vi "App - analyze RUS V6.vi"() -> ()   [LabVIEW 2018] (continued)
"temperature str"="184.42600", "file path"=path "D:/Data/Ultrasound/LSCO/LSCO22__130814c/5_Cooling_2nd_try/September_2014/091614/184.42600K_500_2500_2.10000V_0.00000T_Sep16-2014__15-25-55_001_091614.bin", "last mod"=timestamp(3493740355 s since 1904-01-01), "file name str"="D:\\Data\\Ultrasound\\LSCO\\LSCO22__130814c\\5_Cooling_2nd_try\\September_2014\\091614\\184.42600K_500_2500_2.10000V_0.00000T_Sep16-2014__15-25-55_001_091614.bin", "mod time(min)"=58229005.916666664, "file format"=enum."binary", "power(V)"=2.1, "Magn Field(T) "=0.0}, {"temperature"=184.132, "temperature str"="184.13200", "file path"=path "D:/Data/Ultrasound/LSCO/LSCO22__130814c/5_Cooling_2nd_try/September_2014/091614/184.13200K_500_2500_2.10000V_0.00000T_Sep16-2014__15-27-14_001_091614.bin", "last mod"=timestamp(3493740434 s since 1904-01-01), "file name str"="D:\\Data\\Ultrasound\\LSCO\\LSCO22__130814c\\5_Cooling_2nd_try\\September_2014\\091614\\184.13200K_500_2500_2.10000V_0.00000T_Sep16-2014__15-27-14_001_091614.bin", "mod time(min)"=58229007.233333334, "file format"=enum."binary", "power(V)"=2.1, "Magn Field(T) "=0.0}, {"temperature"=183.85, "temperature str"="183.85000", "file path"=path "D:/Data/Ultrasound/LSCO/LSCO22__130814c/5_Cooling_2nd_try/September_2014/091614/183.85000K_500_2500_2.10000V_0.00000T_Sep16-2014__15-28-33_001_091614.bin", "last mod"=timestamp(3493740513 s since 1904-01-01), "file name str"="D:\\Data\\Ultrasound\\LSCO\\LSCO22__130814c\\5_Cooling_2nd_try\\September_2014\\091614\\183.85000K_500_2500_2.10000V_0.00000T_Sep16-2014__15-28-33_001_091614.bin", "mod time(min)"=58229008.55, "file format"=enum."binary", "power(V)"=2.1, "Magn Field(T) "=0.0}, {"temperature"=183.537, "temperature str"="183.53700", "file path"=path "D:/Data/Ultrasound/LSCO/LSCO22__130814c/5_Cooling_2nd_try/September_2014/091614/183.53700K_500_2500_2.10000V_0.00000T_Sep16-2014__15-29-53_001_091614.bin", "last mod"=timestamp(3493740593 s since 1904-01-01), "file name str"="D:\\Data\\Ultrasound\\LSCO\\LSCO22__130814c\\5_Cooling_2nd_try\\September_2014\\091614\\183.53700K_500_2500_2.10000V_0.00000T_Sep16-2014__15-29-53_001_091614.bin", "mod time(min)"=58229009.88333333, "file format"=enum."binary", "power(V)"=2.1, "Magn Field(T) "=0.0}, {"temperature"=183.227, "temperature str"="183.22700", "file path"=path "D:/Data/Ultrasound/LSCO/LSCO22__130814c/5_Cooling_2nd_try/September_2014/091614/183.22700K_500_2500_2.10000V_0.00000T_Sep16-2014__15-31-12_001_091614.bin", "last mod"=timestamp(3493740672 s since 1904-01-01), "file name str"="D:\\Data\\Ultrasound\\LSCO\\LSCO22__130814c\\5_Cooling_2nd_try\\September_2014\\091614\\183.22700K_500_2500_2.10000V_0.00000T_Sep16-2014__15-31-12_001_091614.bin", "mod time(min)"=58229011.2, "file format"=enum."binary", "power(V)"=2.1, "Magn Field(T) "=0.0}, {"temperature"=182.898, "temperature str"="182.89800", "file path"=path "D:/Data/Ultrasound/LSCO/LSCO22__130814c/5_Cooling_2nd_try/September_2014/091614/182.89800K_500_2500_2.10000V_0.00000T_Sep16-2014__15-32-31_001_091614.bin", "last mod"=timestamp(3493740751 s since 1904-01-01), "file name str"="D:\\Data\\Ultrasound\\LSCO\\LSCO22__130814c\\5_Cooling_2nd_try\\September_2014\\091614\\182.89800K_500_2500_2.10000V_0.00000T_Sep16-2014__15-32-31_001_091614.bin", "mod time(min)"=58229012.516666666, "file format"=enum."binary", "power(V)"=2.1, "Magn Field(T) "=0.0}, {"temperature"=182.567, "temperature str"="182.56700", "file path"=path "D:/Data/Ultrasound/LSCO/LSCO22__130814c/5_Cooling_2nd_try/September_2014/091614/182.56700K_500_2500_2.10000V_0.00000T_Sep16-2014__15-33-51_001_091614.bin", "last mod"=timestamp(3493740831 s since 1904-01-01), "file name str"="D:\\Data\\Ultrasound\\LSCO\\LSCO22__130814c\\5_Cooling_2nd_try\\September_2014\\091614\\182.56700K_500_2500_2.10000V_0.00000T_Sep16-2014__15-33-51_001_091614.bin", "mod time(min)"=58229013.85, "file format"=enum."binary", "power(V)"=2.1, "Magn Field(T) "=0.0}, {"temperature"=182.25, "temperature str"="182.25000", "file path"=path "D:/Data/Ultrasound/LSCO/LSCO22__130814c/5_Cooling_2nd_try/September_2014/091614/182.25000K_500_2500_2.10000V_0.00000T_Sep16-2014__15-35-10_001_091614.bin", "last mod"=timestamp(3493740910 s since 1904-01-01), "file name str"="D:\\Data\\Ultrasound\\LSCO\\LSCO22__130814c\\5_Cooling_2nd_try\\September_2014\\091614\\182.25000K_500_2500_2.10000V_0.00000T_Sep16-2014__15-35-10_001_091614.bin", "mod time(min)"=58229015.166666664, "file format"=enum."binary", "power(V)"=2.1, "Magn Field(T) "=0.0}, {"temperature"=181.923, "temperature str"="181.92300", "file path"=path "D:/Data/Ultrasound/LSCO/LSCO22__130814c/5_Cooling_2nd_try/September_2014/091614/181.92300K_500_2500_2.10000V_0.00000T_Sep16-2014__15-36-30_001_091614.bin", "last mod"=timestamp(3493740990 s since 1904-01-01), "file name str"="D:\\Data\\Ultrasound\\LSCO\\LSCO22__130814c\\5_Cooling_2nd_try\\September_2014\\091614\\181.92300K_500_2500_2.10000V_0.00000T_Sep16-2014__15-36-30_001_091614.bin", "mod time(min)"=58229016.5, "file format"=enum."binary", "power(V)"=2.1, "Magn Field(T) "=0.0}, {"temperature"=181.605, "temperature str"="181.60500", "file path"=path "D:/Data/Ultrasound/LSCO/LSCO22__130814c/5_Cooling_2nd_try/September_2014/091614/181.60500K_500_2500_2.10000V_0.00000T_Sep16-2014__15-37-49_001_091614.bin", "last mod"=timestamp(3493741069 s since 1904-01-01), "file name str"="D:\\Data\\Ultrasound\\LSCO\\LSCO22__130814c\\5_Cooling_2nd_try\\September_2014\\091614\\181.60500K_500_2500_2.10000V_0.00000T_Sep16-2014__15-37-49_001_091614.bin", "mod time(min)"=58229017.81666667, "file format"=enum."binary", "power(V)"=2.1, "Magn Field(T) "=0.0}, {"temperature"=181.283, "temperature str"="181.28300", "file path"=path "D:/Data/Ultrasound/LSCO/LSCO22__130814c/5_Cooling_2nd_try/September_2014/091614/181.28300K_500_2500_2.10000V_0.00000T_Sep16-2014__15-39-08_001_091614.bin", "last mod"=timestamp(3493741148 s since 1904-01-01), "file name str"="D:\\Data\\Ultrasound\\LSCO\\LSCO22__130814c\\5_Cooling_2nd_try\\September_2014\\091614\\181.28300K_500_2500_2.10000V_0.00000T_Sep16-2014__15-39-08_001_091614.bin", "mod time(min)"=58229019.13333333, "file format"=enum."binary", "power(V)"=2.1, "Magn Field(T) "=0.0}, {"temperature"=180.967, "temperature str"="180.96700", "file path"=path "D:/Data/Ultrasound/LSCO/LSCO22__130814c/5_Cooling_2nd_try/September_2014/091614/180.96700K_500_2500_2.10000V_0.00000T_Sep16-2014__15-40-28_001_091614.bin", "last mod"=timestamp(3493741228 s since 1904-01-01), "file name str"="D:\\Data\\Ultrasound\\LSCO\\LSCO22__130814c\\5_Cooling_2nd_try\\September_2014\\091614\\180.96700K_500_2500_2.10000V_0.00000T_Sep16-2014__15-40-28_001_091614.bin", "mod time(min)"=58229020.46666667, "file format"=enum."binary", "power(V)"=2.1, "Magn Field(T) "=0.0}, {"temperature"=180.662, "temperature str"="180.66200", "file path"=path "D:/Data/Ultrasound/LSCO/LSCO22__130814c/5_Cooling_2nd_try/September_2014/091614/180.66200K_500_2500_2.10000V_0.00000T_Sep16-2014__15-41-47_001_091614.bin", "last mod"=timestamp(3493741307 s since 1904-01-01), "file name str"="D:\\Data\\Ultrasound\\LSCO\\LSCO22__130814c\\5_Cooling_2nd_try\\September_2014\\091614\\180.66200K_500_2500_2.10000V_0.00000T_Sep16-2014__15-41-47_001_091614.bin", "mod time(min)"=58229021.78333333, "file format"=enum."binary", "power(V)"=2.1, "Magn Field(T) "=0.0}, {"temperature"=180.335, "temperature str"="180.33500", "file path"=path "D:/Data/Ultrasound/LSCO/LSCO22__130814c/5_Cooling_2nd_try/September_2014/091614/180.33500K_500_2500_2.10000V_0.00000T_Sep16-2014__15-43-06_001_091614.bin", "last mod"=timestamp(3493741386 s since 1904-01-01), "file name str"="D:\\Data\\Ultrasound\\LSCO\\LSCO22__130814c\\5_Cooling_2nd_try\\September_2014\\091614\\180.33500K_500_2500_2.10000V_0.00000T_Sep16-2014__15-43-06_001_091614.bin", "mod time(min)"=58229023.1, "file format"=enum."binary", "power(V)"=2.1, "Magn Field(T) "=0.0}, {"temperature"=180.012, "temperature str"="180.01200", "file path"=path "D:/Data/Ultrasound/LSCO/LSCO22__130814c/5_Cooling_2nd_try/September_2014/091614/180.01200K_500_2500_2.10000V_0.00000T_Sep16-2014__15-44-26_001_091614.bin", "last mod"=timestamp(3493741466 s since 1904-01-01), "file name str"="D:\\Data\\Ultrasound\\LSCO\\LSCO22__130814c\\5_Cooling_2nd_try\\September_2014\\091614\\180.01200K_500_2500_2.10000V_0.00000T_Sep16-2014__15-44-26_001_091614.bin", "mod time(min)"=58229024.43333333, "file format"=enum."binary", "power(V)"=2.1, "Magn Field(T) "=0.0}, {"temperature"=179.664, "temperature str"="179.66400", "file path"=path "D:/Data/Ultrasound/LSCO/LSCO22__130814c/5_Cooling_2nd_try/September_2014/091614/179.66400K_500_2500_2.10000V_0.00000T_Sep16-2014__15-45-45_001_091614.bin", "last mod"=timestamp(3493741545 s since 1904-01-01), "file name str"="D:\\Data\\Ultrasound\\LSCO\\LSCO22__130814c\\5_Cooling_2nd_try\\September_2014\\091614\\179.66400K_500_2500_2.10000V_0.00000T_Sep16-2014__15-45-45_001_091614.bin", "mod time(min)"=58229025.75, "file format"=enum."binary", "power(V)"=2.1, "Magn Field(T) "=0.0}, {"temperature"=179.311, "temperature str"="179.31100", "file path"=path "D:/Data/Ultrasound/LSCO/LSCO22__130814c/5_Cooling_2nd_try/September_2014/091614/179.31100K_500_2500_2.10000V_0.00000T_Sep16-2014__15-47-05_001_091614.bin", "last mod"=timestamp(3493741625 s since 1904-01-01), "file name str"="D:\\Data\\Ultrasound\\LSCO\\LSCO22__130814c\\5_Cooling_2nd_try\\September_2014\\091614\\179.31100K_500_2500_2.10000V_0.00000T_Sep16-2014__15-47-05_001_091614.bin", "mod time(min)"=58229027.083333336, "file format"=enum."binary", "power(V)"=2.1, "Magn Field(T) "=0.0}, {"temperature"=178.96, "temperature str"="178.96000", "file path"=path "D:/Data/Ultrasound/LSCO/LSCO22__130814c/5_Cooling_2nd_try/September_2014/091614/178.96000K_500_2500_2.10000V_0.00000T_Sep16-2014__15-48-24_001_091614.bin", "last mod"=timestamp(3493741704 s since 1904-01-01), "file name str"="D:\\Data\\Ultrasound\\LSCO\\LSCO22__130814c\\5_Cooling_2nd_try\\September_2014\\091614\\178.96000K_500_2500_2.10000V_0.00000T_Sep16-2014__15-48-24_001_091614.bin", "mod time(min)"=58229028.4, "file format"=enum."binary", "power(V)"=2.1, "Magn Field(T) "=0.0}, {"temperature"=178.579, "temperature str"="178.57900", "file path"=path "D:/Data/Ultrasound/LSCO/LSCO22__130814c/5_Cooling_2nd_try/September_2014/091614/178.57900K_500_2500_2.10000V_0.00000T_Sep16-2014__15-49-43_001_091614.bin", "last mod"=timestamp(3493741783 s since 1904-01-01), "file name str"="D:\\Data\\Ultrasound\\LSCO\\LSCO22__130814c\\5_Cooling_2nd_try\\September_2014\\091614\\178.57900K_500_2500_2.10000V_0.00000T_Sep16-2014__15-49-43_001_091614.bin", "mod time(min)"=58229029.71666667, "file format"=enum."binary", "power(V)"=2.1, "Magn Field(T) "=0.0}, {"temperature"=178.21, "temperature str"="178.21000", "file path"=path "D:/Data/Ultrasound/LSCO/LSCO22__130814c/5_Cooling_2nd_try/September_2014/091614/178.21000K_500_2500_2.10000V_0.00000T_Sep16-2014__15-51-03_001_091614.bin", "last mod"=timestamp(3493741863 s since 1904-01-01), "file name str"="D:\\Data\\Ultrasound\\LSCO\\LSCO22__130814c\\5_Cooling_2nd_try\\September_2014\\091614\\178.21000K_500_2500_2.10000V_0.00000T_Sep16-2014__15-51-03_001_091614.bin", "mod time(min)"=58229031.05, "file format"=enum."binary", "power(V)"=2.1, "Magn Field(T) "=0.0}, {"temperature"=177.848, "temperature str"="177.84800", "file path"=path "D:/Data/Ultrasound/LSCO/LSCO22__130814c/5_Cooling_2nd_try/September_2014/091614/177.84800K_500_2500_2.10000V_0.00000T_Sep16-2014__15-52-22_001_091614.bin", "last mod"=timestamp(3493741942 s since 1904-01-01), "file name str"="D:\\Data\\Ultrasound\\LSCO\\LSCO22__130814c\\5_Cooling_2nd_try\\September_2014\\091614\\177.84800K_500_2500_2.10000V_0.00000T_Sep16-2014__15-52-22_001_091614.bin", "mod time(min)"=58229032.36666667, "file format"=enum."binary", "power(V)"=2.1, "Magn Field(T) "=0.0}, {"temperature"=177.556, "temperature str"="177.55600", "file path"=path "D:/Data/Ultrasound/LSCO/LSCO22__130814c/5_Cooling_2nd_try/September_2014/091614/177.55600K_500_2500_2.10000V_0.00000T_Sep16-2014__15-53-41_001_091614.bin", "last mod"=timestamp(3493742021 s since 1904-01-01), "file name str"="D:\\Data\\Ultrasound\\LSCO\\LSCO22__130814c\\5_Cooling_2nd_try\\September_2014\\091614\\177.55600K_500_2500_2.10000V_0.00000T_Sep16-2014__15-53-41_001_091614.bin", "mod time(min)"=58229033.68333333, "file format"=enum."binary", "power(V)"=2.1, "Magn Field(T) "=0.0}, {"temperature"=177.306, "temperature str"="177.30600", "file path"=path "D:/Data/Ultrasound/LSCO/LSCO22__130814c/5_Cooling_2nd_try/September_2014/091614/177.30600K_500_2500_2.10000V_0.00000T_Sep16-2014__15-55-01_001_091614.bin", "last mod"=timestamp(3493742101 s since 1904-01-01), "file name str"="D:\\Data\\Ultrasound\\LSCO\\LSCO22__130814c\\5_Cooling_2nd_try\\September_2014\\091614\\177.30600K_500_2500_2.10000V_0.00000T_Sep16-2014__15-55-01_001_091614.bin", "mod time(min)"=58229035.016666666, "file format"=enum."binary", "power(V)"=2.1, "Magn Field(T) "=0.0}, {"temperature"=177.009, "temperature str"="177.00900", "file path"=path "D:/Data/Ultrasound/LSCO/LSCO22__130814c/5_Cooling_2nd_try/September_2014/091614/177.00900K_500_2500_2.10000V_0.00000T_Sep16-2014__15-56-20_001_091614.bin", "last mod"=timestamp(3493742180 s since 1904-01-01), "file name str"="D:\\Data\\Ultrasound\\LSCO\\LSCO22__130814c\\5_Cooling_2nd_try\\September_2014\\091614\\177.00900K_500_2500_2.10000V_0.00000T_Sep16-2014__15-56-20_001_091614.bin", "mod time(min)"=58229036.333333336, "file format"=enum."binary", "power(V)"=2.1, "Magn Field(T) "=0.0}, {"temperature"=176.677, "temperature str"="176.67700", "file path"=path "D:/Data/Ultrasound/LSCO/LSCO22__130814c/5_Cooling_2nd_try/September_2014/091614/176.67700K_500_2500_2.10000V_0.00000T_Sep16-2014__15-57-39_001_091614.bin", "last mod"=timestamp(3493742259 s since 1904-01-01), "file name str"="D:\\Data\\Ultrasound\\LSCO\\LSCO22__130814c\\5_Cooling_2nd_try\\September_2014\\091614\\176.67700K_500_2500_2.10000V_0.00000T_Sep16-2014__15-57-39_001_091614.bin", "mod time(min)"=58229037.65, "file format"=enum."binary", "power(V)"=2.1, "Magn Field(T) "=0.0}, {"temperature"=176.315, "temperature str"="176.31500", "file path"=path "D:/Data/Ultrasound/LSCO/LSCO22__130814c/5_Cooling_2nd_try/September_2014/091614/176.31500K_500_2500_2.10000V_0.00000T_Sep16-2014__15-58-59_001_091614.bin", "last mod"=timestamp(3493742339 s since 1904-01-01), "file name str"="D:\\Data\\Ultrasound\\LSCO\\LSCO22__130814c\\5_Cooling_2nd_try\\September_2014\\091614\\176.31500K_500_2500_2.10000V_0.00000T_Sep16-2014__15-58-59_001_091614.bin", "mod time(min)"=58229038.983333334, "file format"=enum."binary", "power(V)"=2.1, "Magn Field(T) "=0.0}, {"temperature"=175.963, "temperature str"="175.96300", "file path"=path "D:/Data/Ultrasound/LSCO/LSCO22__130814c/5_Cooling_2nd_try/September_2014/091614/175.96300K_500_2500_2.10000V_0.00000T_Sep16-2014__16-00-18_001_091614.bin", "last mod"=timestamp(3493742418 s since 1904-01-01), "file name str"="D:\\Data\\Ultrasound\\LSCO\\LSCO22__130814c\\5_Cooling_2nd_try\\September_2014\\091614\\175.96300K_500_2500_2.10000V_0.00000T_Sep16-2014__16-00-18_001_091614.bin", "mod time(min)"=58229040.3, "file format"=enum."binary", "power(V)"=2.1, "Magn Field(T) "=0.0}, {"temperature"=175.634, "temperature str"="175.63400", "file path"=path "D:/Data/Ultrasound/LSCO/LSCO22__130814c/5_Cooling_2nd_try/September_2014/091614/175.63400K_500_2500_2.10000V_0.00000T_Sep16-2014__16-01-37_001_091614.bin", "last mod"=timestamp(3493742497 s since 1904-01-01), "file name str"="D:\\Data\\Ultrasound\\LSCO\\LSCO22__130814c\\5_Cooling_2nd_try\\September_2014\\091614\\175.63400K_500_2500_2.10000V_0.00000T_Sep16-2014__16-01-37_001_091614.bin", "mod time(min)"=58229041.61666667, "file format"=enum."binary", "power(V)"=2.1, "Magn Field(T) "=0.0}, {"temperature"=175.302, "temperature str"="175.30200", "file path"=path "D:/Data/Ultrasound/LSCO/LSCO22__130814c/5_Cooling_2nd_try/September_2014/091614/175.30200K_500_2500_2.10000V_0.00000T_Sep16-2014__16-02-57_001_091614.bin", "last mod"=timestamp(3493742577 s since 1904-01-01), "file name str"="D:\\Data\\Ultrasound\\LSCO\\LSCO22__130814c\\5_Cooling_2nd_try\\September_2014\\091614\\175.30200K_500_2500_2.10000V_0.00000T_Sep16-2014__16-02-57_001_091614.bin", "mod time(min)"=58229042.95, "file format"=enum."binary", "power(V)"=2.1, "Magn Field(T) "=0.0}, {"temperature"=174.985, "temperature str"="174.98500", "file path"=path "D:/Data/Ultrasound/LSCO/LSCO22__130814c/5_Cooling_2nd_try/September_2014/091614/174.98500K_500_2500_2.10000V_0.00000T_Sep16-2014__16-04-16_001_091614.bin", "last mod"=timestamp(3493742656 s since 1904-01-01), "file name str"="D:\\Data\\Ultrasound\\LSCO\\LSCO22__130814c\\5_Cooling_2nd_try\\September_2014\\091614\\174.98500K_500_2500_2.10000V_0.00000T_Sep16-2014__16-04-16_001_091614.bin", "mod time(min)"=58229044.266666666, "file format"=enum."binary", "power(V)"=2.1, "Magn Field(T) "=0.0}, {"temperature"=174.654, "temperature str"="174.65400", "file path"=path "D:/Data/Ultrasound/LSCO/LSCO22__130814c/5_Cooling_2nd_try/September_2014/091614/174.65400K_500_2500_2.10000V_0.00000T_Sep16-2014__16-05-35_001_091614.bin", "last mod"=timestamp(3493742735 s since 1904-01-01), "file name str"="D:\\Data\\Ultrasound\\LSCO\\LSCO22__130814c\\5_Cooling_2nd_try\\September_2014\\091614\\174.65400K_500_2500_2.10000V_0.00000T_Sep16-2014__16-05-35_001_091614.bin", "mod time(min)"=58229045.583333336, "file format"=enum."binary", "power(V)"=2.1, "Magn Field(T) "=0.0}, {"temperature"=174.316, "temperature str"="174.31600", "file path"=path "D:/Data/Ultrasound/LSCO/LSCO22__130814c/5_Cooling_2nd_try/September_2014/091614/174.31600K_500_2500_2.10000V_0.00000T_Sep16-2014__16-06-55_001_091614.bin", "last mod"=timestamp(3493742815 s since 1904-01-01), "file name str"="D:\\Data\\Ultrasound\\LSCO\\LSCO22__130814c\\5_Cooling_2nd_try\\September_2014\\091614\\174.31600K_500_2500_2.10000V_0.00000T_Sep16-2014__16-06-55_001_091614.bin", "mod time(min)"=58229046.916666664, "file format"=enum."binary", "power(V)"=2.1, "Magn Field(T) "=0.0}, {"temperature"=173.984, "temperature str"="173.98400", "file path"=path "D:/Data/Ultrasound/LSCO/LSCO22__130814c/5_Cooling_2nd_try/September_2014/091614/173.98400K_500_2500_2.10000V_0.00000T_Sep16-2014__16-08-14_001_091614.bin", "last mod"=timestamp(3493742894 s since 1904-01-01), "file name str"="D:\\Data\\Ultrasound\\LSCO\\LSCO22__130814c\\5_Cooling_2nd_try\\September_2014\\091614\\173.98400K_500_2500_2.10000V_0.00000T_Sep16-2014__16-08-14_001_091614.bin", "mod time(min)"=58229048.233333334, "file format"=enum."binary", "power(V)"=2.1, "Magn Field(T) "=0.0}, {"temperature"=173.642, "temperature str"="173.64200", "file path"=path "D:/Data/Ultrasound/LSCO/LSCO22__130814c/5_Cooling_2nd_try/September_2014/091614/173.64200K_500_2500_2.10000V_0.00000T_Sep16-2014__16-09-33_001_091614.bin", "last mod"=timestamp(3493742973 s since 1904-01-01), "file name str"="D:\\Data\\Ultrasound\\LSCO\\LSCO22__130814c\\5_Cooling_2nd_try\\September_2014\\091614\\173.64200K_500_2500_2.10000V_0.00000T_Sep16-2014__16-09-33_001_091614.bin", "mod time(min)"=58229049.55, "file format"=enum."binary", "power(V)"=2.1, "Magn Field(T) "=0.0}, {"temperature"=173.314, "temperature str"="173.31400", "file path"=path "D:/Data/Ultrasound/LSCO/LSCO22__130814c/5_Cooling_2nd_try/September_2014/091614/173.31400K_500_2500_2.10000V_0.00000T_Sep16-2014__16-10-53_001_091614.bin", "last mod"=timestamp(3493743053 s since 1904-01-01), "file name str"="D:\\Data\\Ultrasound\\LSCO\\LSCO22__130814c\\5_Cooling_2nd_try\\September_2014\\091614\\173.31400K_500_2500_2.10000V_0.00000T_Sep16-2014__16-10-53_001_091614.bin", "mod time(min)"=58229050.88333333, "file format"=enum."binary", "power(V)"=2.1, "Magn Field(T) "=0.0}, {"temperature"=172.974, "temperature str"="172.97400", "file path"=path "D:/Data/Ultrasound/LSCO/LSCO22__130814c/5_Cooling_2nd_try/September_2014/091614/172.97400K_500_2500_2.10000V_0.00000T_Sep16-2014__16-12-12_001_091614.bin", "last mod"=timestamp(3493743132 s since 1904-01-01), "file name str"="D:\\Data\\Ultrasound\\LSCO\\LSCO22__130814c\\5_Cooling_2nd_try\\September_2014\\091614\\172.97400K_500_2500_2.10000V_0.00000T_Sep16-2014__16-12-12_001_091614.bin", "mod time(min)"=58229052.2, "file format"=enum."binary", "power(V)"=2.1, "Magn Field(T) "=0.0}, {"temperature"=172.632, "temperature str"="172.63200", "file path"=path "D:/Data/Ultrasound/LSCO/LSCO22__130814c/5_Cooling_2nd_try/September_2014/091614/172.63200K_500_2500_2.10000V_0.00000T_Sep16-2014__16-13-31_001_091614.bin", "last mod"=timestamp(3493743211 s since 1904-01-01), "file name str"="D:\\Data\\Ultrasound\\LSCO\\LSCO22__130814c\\5_Cooling_2nd_try\\September_2014\\091614\\172.63200K_500_2500_2.10000V_0.00000T_Sep16-2014__16-13-31_001_091614.bin", "mod time(min)"=58229053.516666666, "file format"=enum."binary", "power(V)"=2.1, "Magn Field(T) "=0.0}, {"temperature"=172.303, "temperature str"="172.30300", "file path"=path "D:/Data/Ultrasound/LSCO/LSCO22__130814c/5_Cooling_2nd_try/September_2014/091614/172.30300K_500_2500_2.10000V_0.00000T_Sep16-2014__16-14-51_001_091614.bin", "last mod"=timestamp(3493743291 s since 1904-01-01), "file name str"="D:\\Data\\Ultrasound\\LSCO\\LSCO22__130814c\\5_Cooling_2nd_try\\September_2014\\091614\\172.30300K_500_2500_2.10000V_0.00000T_Sep16-2014__16-14-51_001_091614.bin", "mod time(min)"=58229054.85, "file format"=enum."binary", "power(V)"=2.1, "Magn Field(T) "=0.0}, {"temperature"=171.947, "temperature str"="171.94700", "file path"=path "D:/Data/Ultrasound/LSCO/LSCO22__130814c/5_Cooling_2nd_try/September_2014/091614/171.94700K_500_2500_2.10000V_0.00000T_Sep16-2014__16-16-10_001_091614.bin", "last mod"=timestamp(3493743370 s since 1904-01-01), "file name str"="D:\\Data\\Ultrasound\\LSCO\\LSCO22__130814c\\5_Cooling_2nd_try\\September_2014\\091614\\171.94700K_500_2500_2.10000V_0.00000T_Sep16-2014__16-16-10_001_091614.bin", "mod time(min)"=58229056.166666664, "file format"=enum."binary", "power(V)"=2.1, "Magn Field(T) "=0.0}, {"temperature"=171.593, "temperature str"="171.59300", "file path"=path "D:/Data/Ultrasound/LSCO/LSCO22__130814c/5_Cooling_2nd_try/September_2014/091614/171.59300K_500_2500_2.10000V_0.00000T_Sep16-2014__16-17-29_001_091614.bin", "last mod"=timestamp(3493743449 s since 1904-01-01), "file name str"="D:\\Data\\Ultrasound\\LSCO\\LSCO22__130814c\\5_Cooling_2nd_try\\September_2014\\091614\\171.59300K_500_2500_2.10000V_0.00000T_Sep16-2014__16-17-29_001_091614.bin", "mod time(min)"=58229057.483333334, "file format"=enum."binary", "power(V)"=2.1, "Magn Field(T) "=0.0}, {"temperature"=171.216, "temperature str"="171.21600", "file path"=path "D:/Data/Ultrasound/LSCO/LSCO22__130814c/5_Cooling_2nd_try/September_2014/091614/171.21600K_500_2500_2.10000V_0.00000T_Sep16-2014__16-18-49_001_091614.bin", "last mod"=timestamp(3493743529 s since 1904-01-01), "file name str"="D:\\Data\\Ultrasound\\LSCO\\LSCO22__130814c\\5_Cooling_2nd_try\\September_2014\\091614\\171.21600K_500_2500_2.10000V_0.00000T_Sep16-2014__16-18-49_001_091614.bin", "mod time(min)"=58229058.81666667, "file format"=enum."binary", "power(V)"=2.1, "Magn Field(T) "=0.0}, {"temperature"=170.839, "temperature str"="170.83900", "file path"=path "D:/Data/Ultrasound/LSCO/LSCO22__130814c/5_Cooling_2nd_try/September_2014/091614/170.83900K_500_2500_2.10000V_0.00000T_Sep16-2014__16-20-08_001_091614.bin", "last mod"=timestamp(3493743608 s since 1904-01-01), "file name str"="D:\\Data\\Ultrasound\\LSCO\\LSCO22__130814c\\5_Cooling_2nd_try\\September_2014\\091614\\170.83900K_500_2500_2.10000V_0.00000T_Sep16-2014__16-20-08_001_091614.bin", "mod time(min)"=58229060.13333333, "file format"=enum."binary", "power(V)"=2.1, "Magn Field(T) "=0.0}, {"temperature"=170.496, "temperature str"="170.49600", "file path"=path "D:/Data/Ultrasound/LSCO/LSCO22__130814c/5_Cooling_2nd_try/September_2014/091614/170.49600K_500_2500_2.10000V_0.00000T_Sep16-2014__16-21-28_001_091614.bin", "last mod"=timestamp(3493743688 s since 1904-01-01), "file name str"="D:\\Data\\Ultrasound\\LSCO\\LSCO22__130814c\\5_Cooling_2nd_try\\September_2014\\091614\\170.49600K_500_2500_2.10000V_0.00000T_Sep16-2014__16-21-28_001_091614.bin", "mod time(min)"=58229061.46666667, "file format"=enum."binary", "power(V)"=2.1, "Magn Field(T) "=0.0}, {"temperature"=170.187, "temperature str"="170.18700", "file path"=path "D:/Data/Ultrasound/LSCO/LSCO22__130814c/5_Cooling_2nd_try/September_2014/091614/170.18700K_500_2500_2.10000V_0.00000T_Sep16-2014__16-22-47_001_091614.bin", "last mod"=timestamp(3493743767 s since 1904-01-01), "file name str"="D:\\Data\\Ultrasound\\LSCO\\LSCO22__130814c\\5_Cooling_2nd_try\\September_2014\\091614\\170.18700K_500_2500_2.10000V_0.00000T_Sep16-2014__16-22-47_001_091614.bin", "mod time(min)"=58229062.78333333, "file format"=enum."binary", "power(V)"=2.1, "Magn Field(T) "=0.0}, {"temperature"=169.921, "temperature str"="169.92100", "file path"=path "D:/Data/Ultrasound/LSCO/LSCO22__130814c/5_Cooling_2nd_try/September_2014/091614/169.92100K_500_2500_2.10000V_0.00000T_Sep16-2014__16-24-06_001_091614.bin", "last mod"=timestamp(3493743846 s since 1904-01-01), "file name str"="D:\\Data\\Ultrasound\\LSCO\\LSCO22__130814c\\5_Cooling_2nd_try\\September_2014\\091614\\169.92100K_500_2500_2.10000V_0.00000T_Sep16-2014__16-24-06_001_091614.bin", "mod time(min)"=58229064.1, "file format"=enum."binary", "power(V)"=2.1, "Magn Field(T) "=0.0}, {"temperature"=169.62, "temperature str"="169.62000", "file path"=path "D:/Data/Ultrasound/LSCO/LSCO22__130814c/5_Cooling_2nd_try/September_2014/091614/169.62000K_500_2500_2.10000V_0.00000T_Sep16-2014__16-25-26_001_091614.bin", "last mod"=timestamp(3493743926 s since 1904-01-01), "file name str"="D:\\Data\\Ultrasound\\LSCO\\LSCO22__130814c\\5_Cooling_2nd_try\\September_2014\\091614\\169.62000K_500_2500_2.10000V_0.00000T_Sep16-2014__16-25-26_001_091614.bin", "mod time(min)"=58229065.43333333, "file format"=enum."binary", "power(V)"=2.1, "Magn Field(T) "=0.0}, {"temperature"=169.281, "temperature str"="169.28100", "file path"=path "D:/Data/Ultrasound/LSCO/LSCO22__130814c/5_Cooling_2nd_try/September_2014/091614/169.28100K_500_2500_2.10000V_0.00000T_Sep16-2014__16-26-45_001_091614.bin", "last mod"=timestamp(3493744005 s since 1904-01-01), "file name str"="D:\\Data\\Ultrasound\\LSCO\\LSCO22__130814c\\5_Cooling_2nd_try\\September_2014\\091614\\169.28100K_500_2500_2.10000V_0.00000T_Sep16-2014__16-26-45_001_091614.bin", "mod time(min)"=58229066.75, "file format"=enum."binary", "power(V)"=2.1, "Magn Field(T) "=0.0}, {"temperature"=168.934, "temperature str"="168.93400", "file path"=path "D:/Data/Ultrasound/LSCO/LSCO22__130814c/5_Cooling_2nd_try/September_2014/091614/168.93400K_500_2500_2.10000V_0.00000T_Sep16-2014__16-28-04_001_091614.bin", "last mod"=timestamp(3493744084 s since 1904-01-01), "file name str"="D:\\Data\\Ultrasound\\LSCO\\LSCO22__130814c\\5_Cooling_2nd_try\\September_2014\\091614\\168.93400K_500_2500_2.10000V_0.00000T_Sep16-2014__16-28-04_001_091614.bin", "mod time(min)"=58229068.06666667, "file format"=enum."binary", "power(V)"=2.1, "Magn Field(T) "=0.0}, {"temperature"=168.567, "temperature str"="168.56700", "file path"=path "D:/Data/Ultrasound/LSCO/LSCO22__130814c/5_Cooling_2nd_try/September_2014/091614/168.56700K_500_2500_2.10000V_0.00000T_Sep16-2014__16-29-24_001_091614.bin", "last mod"=timestamp(3493744164 s since 1904-01-01), "file name str"="D:\\Data\\Ultrasound\\LSCO\\LSCO22__130814c\\5_Cooling_2nd_try\\September_2014\\091614\\168.56700K_500_2500_2.10000V_0.00000T_Sep16-2014__16-29-24_001_091614.bin", "mod time(min)"=58229069.4, "file format"=enum."binary", "power(V)"=2.1, "Magn Field(T) "=0.0}, {"temperature"=168.198, "temperature str"="168.19800", "file path"=path "D:/Data/Ultrasound/LSCO/LSCO22__130814c/5_Cooling_2nd_try/September_2014/091614/168.19800K_500_2500_2.10000V_0.00000T_Sep16-2014__16-30-43_001_091614.bin", "last mod"=timestamp(3493744243 s since 1904-01-01), "file name str"="D:\\Data\\Ultrasound\\LSCO\\LSCO22__130814c\\5_Cooling_2nd_try\\September_2014\\091614\\168.19800K_500_2500_2.10000V_0.00000T_Sep16-2014__16-30-43_001_091614.bin", "mod time(min)"=58229070.71666667, "file format"=enum."binary", "power(V)"=2.1, "Magn Field(T) "=0.0}, {"temperature"=166.235, "temperature str"="166.23500", "file path"=path "D:/Data/Ultrasound/LSCO/LSCO22__130814c/5_Cooling_2nd_try/September_2014/091614/166.23500K_500_2500_2.10000V_0.00000T_Sep16-2014__16-32-02_001_091614.bin", "last mod"=timestamp(3493744322 s since 1904-01-01), "file name str"="D:\\Data\\Ultrasound\\LSCO\\LSCO22__130814c\\5_Cooling_2nd_try\\September_2014\\091614\\166.23500K_500_2500_2.10000V_0.00000T_Sep16-2014__16-32-02_001_091614.bin", "mod time(min)"=58229072.03333333, "file format"=enum."binary", "power(V)"=2.1, "Magn Field(T) "=0.0}, {"temperature"=167.465, "temperature str"="167.46500", "file path"=path "D:/Data/Ultrasound/LSCO/LSCO22__130814c/5_Cooling_2nd_try/September_2014/091614/167.46500K_500_2500_2.10000V_0.00000T_Sep16-2014__16-33-22_001_091614.bin", "last mod"=timestamp(3493744402 s since 1904-01-01), "file name str"="D:\\Data\\Ultrasound\\LSCO\\LSCO22__130814c\\5_Cooling_2nd_try\\September_2014\\091614\\167.46500K_500_2500_2.10000V_0.00000T_Sep16-2014__16-33-22_001_091614.bin", "mod time(min)"=58229073.36666667, "file format"=enum."binary", "power(V)"=2.1, "Magn Field(T) "=0.0}, {"temperature"=167.68, "temperature str"="167.68000", "file path"=path "D:/Data/Ultrasound/LSCO/LSCO22__130814c/5_Cooling_2nd_try/September_2014/091614/167.68000K_500_2500_2.10000V_0.00000T_Sep16-2014__16-34-41_001_091614.bin", "last mod"=timestamp(3493744481 s since 1904-01-01), "file name str"="D:\\Data\\Ultrasound\\LSCO\\LSCO22__130814c\\5_Cooling_2nd_try\\September_2014\\091614\\167.68000K_500_2500_2.10000V_0.00000T_Sep16-2014__16-34-41_001_091614.bin", "mod time(min)"=58229074.68333333, "file format"=enum."binary", "power(V)"=2.1, "Magn Field(T) "=0.0}, {"temperature"=166.454, "temperature str"="166.45400", "file path"=path "D:/Data/Ultrasound/LSCO/LSCO22__130814c/5_Cooling_2nd_try/September_2014/091614/166.45400K_500_2500_2.10000V_0.00000T_Sep16-2014__16-36-01_001_091614.bin", "last mod"=timestamp(3493744561 s since 1904-01-01), "file name str"="D:\\Data\\Ultrasound\\LSCO\\LSCO22__130814c\\5_Cooling_2nd_try\\September_2014\\091614\\166.45400K_500_2500_2.10000V_0.00000T_Sep16-2014__16-36-01_001_091614.bin", "mod time(min)"=58229076.016666666, "file format"=enum."binary", "power(V)"=2.1, "Magn Field(T) "=0.0}, {"temperature"=166.595, "temperature str"="166.59500", "file path"=path "D:/Data/Ultrasound/LSCO/LSCO22__130814c/5_Cooling_2nd_try/September_2014/091614/166.59500K_500_2500_2.10000V_0.00000T_Sep16-2014__16-37-20_001_091614.bin", "last mod"=timestamp(3493744640 s since 1904-01-01), "file name str"="D:\\Data\\Ultrasound\\LSCO\\LSCO22__130814c\\5_Cooling_2nd_try\\September_2014\\091614\\166.59500K_500_2500_2.10000V_0.00000T_Sep16-2014__16-37-20_001_091614.bin", "mod time(min)"=58229077.333333336, "file format"=enum."binary", "power(V)"=2.1, "Magn Field(T) "=0.0}, {"temperature"=166.194, "temperature str"="166.19400", "file path"=path "D:/Data/Ultrasound/LSCO/LSCO22__130814c/5_Cooling_2nd_try/September_2014/091614/166.19400K_500_2500_2.10000V_0.00000T_Sep16-2014__16-38-39_001_091614.bin", "last mod"=timestamp(3493744719 s since 1904-01-01), "file name str"="D:\\Data\\Ultrasound\\LSCO\\LSCO22__130814c\\5_Cooling_2nd_try\\September_2014\\091614\\166.19400K_500_2500_2.10000V_0.00000T_Sep16-2014__16-38-39_001_091614.bin", "mod time(min)"=58229078.65, "file format"=enum."binary", "power(V)"=2.1, "Magn Field(T) "=0.0}, {"temperature"=165.738, "temperature str"="165.73800", "file path"=path "D:/Data/Ultrasound/LSCO/LSCO22__130814c/5_Cooling_2nd_try/September_2014/091614/165.73800K_500_2500_2.10000V_0.00000T_Sep16-2014__16-39-59_001_091614.bin", "last mod"=timestamp(3493744799 s since 1904-01-01), "file name str"="D:\\Data\\Ultrasound\\LSCO\\LSCO22__130814c\\5_Cooling_2nd_try\\September_2014\\091614\\165.73800K_500_2500_2.10000V_0.00000T_Sep16-2014__16-39-59_001_091614.bin", "mod time(min)"=58229079.983333334, "file format"=enum."binary", "power(V)"=2.1, "Magn Field(T) "=0.0}, {"temperature"=165.506, "temperature str"="165.50600", "file path"=path "D:/Data/Ultrasound/LSCO/LSCO22__130814c/5_Cooling_2nd_try/September_2014/091614/165.50600K_500_2500_2.10000V_0.00000T_Sep16-2014__16-41-18_001_091614.bin", "last mod"=timestamp(3493744878 s since 1904-01-01), "file name str"="D:\\Data\\Ultrasound\\LSCO\\LSCO22__130814c\\5_Cooling_2nd_try\\September_2014\\091614\\165.50600K_500_2500_2.10000V_0.00000T_Sep16-2014__16-41-18_001_091614.bin", "mod time(min)"=58229081.3, "file format"=enum."binary", "power(V)"=2.1, "Magn Field(T) "=0.0}, {"temperature"=165.119, "temperature str"="165.11900", "file path"=path "D:/Data/Ultrasound/LSCO/LSCO22__130814c/5_Cooling_2nd_try/September_2014/091614/165.11900K_500_2500_2.10000V_0.00000T_Sep16-2014__16-42-37_001_091614.bin", "last mod"=timestamp(3493744957 s since 1904-01-01), "file name str"="D:\\Data\\Ultrasound\\LSCO\\LSCO22__130814c\\5_Cooling_2nd_try\\September_2014\\091614\\165.11900K_500_2500_2.10000V_0.00000T_Sep16-2014__16-42-37_001_091614.bin", "mod time(min)"=58229082.61666667, "file format"=enum."binary", "power(V)"=2.1, "Magn Field(T) "=0.0}, {"temperature"=164.781, "temperature str"="164.78100", "file path"=path "D:/Data/Ultrasound/LSCO/LSCO22__130814c/5_Cooling_2nd_try/September_2014/091614/164.78100K_500_2500_2.10000V_0.00000T_Sep16-2014__16-43-57_001_091614.bin", "last mod"=timestamp(3493745037 s since 1904-01-01), "file name str"="D:\\Data\\Ultrasound\\LSCO\\LSCO22__130814c\\5_Cooling_2nd_try\\September_2014\\091614\\164.78100K_500_2500_2.10000V_0.00000T_Sep16-2014__16-43-57_001_091614.bin", "mod time(min)"=58229083.95, "file format"=enum."binary", "power(V)"=2.1, "Magn Field(T) "=0.0}, {"temperature"=164.449, "temperature str"="164.44900", "file path"=path "D:/Data/Ultrasound/LSCO/LSCO22__130814c/5_Cooling_2nd_try/September_2014/091614/164.44900K_500_2500_2.10000V_0.00000T_Sep16-2014__16-45-16_001_091614.bin", "last mod"=timestamp(3493745116 s since 1904-01-01), "file name str"="D:\\Data\\Ultrasound\\LSCO\\LSCO22__130814c\\5_Cooling_2nd_try\\September_2014\\091614\\164.44900K_500_2500_2.10000V_0.00000T_Sep16-2014__16-45-16_001_091614.bin", "mod time(min)"=58229085.266666666, "file format"=enum."binary", "power(V)"=2.1, "Magn Field(T) "=0.0}, {"temperature"=164.092, "temperature str"="164.09200", "file path"=path "D:/Data/Ultrasound/LSCO/LSCO22__130814c/5_Cooling_2nd_try/September_2014/091614/164.09200K_500_2500_2.10000V_0.00000T_Sep16-2014__16-46-36_001_091614.bin", "last mod"=timestamp(3493745196 s since 1904-01-01), "file name str"="D:\\Data\\Ultrasound\\LSCO\\LSCO22__130814c\\5_Cooling_2nd_try\\September_2014\\091614\\164.09200K_500_2500_2.10000V_0.00000T_Sep16-2014__16-46-36_001_091614.bin", "mod time(min)"=58229086.6, "file format"=enum."binary", "power(V)"=2.1, "Magn Field(T) "=0.0}, {"temperature"=163.762, "temperature str"="163.76200", "file path"=path "D:/Data/Ultrasound/LSCO/LSCO22__130814c/5_Cooling_2nd_try/September_2014/091614/163.76200K_500_2500_2.10000V_0.00000T_Sep16-2014__16-47-55_001_091614.bin", "last mod"=timestamp(3493745275 s since 1904-01-01), "file name str"="D:\\Data\\Ultrasound\\LSCO\\LSCO22__130814c\\5_Cooling_2nd_try\\September_2014\\091614\\163.76200K_500_2500_2.10000V_0.00000T_Sep16-2014__16-47-55_001_091614.bin", "mod time(min)"=58229087.916666664, "file format"=enum."binary", "power(V)"=2.1, "Magn Field(T) "=0.0}, {"temperature"=163.413, "temperature str"="163.41300", "file path"=path "D:/Data/Ultrasound/LSCO/LSCO22__130814c/5_Cooling_2nd_try/September_2014/091614/163.41300K_500_2500_2.10000V_0.00000T_Sep16-2014__16-49-14_001_091614.bin", "last mod"=timestamp(3493745354 s since 1904-01-01), "file name str"="D:\\Data\\Ultrasound\\LSCO\\LSCO22__130814c\\5_Cooling_2nd_try\\September_2014\\091614\\163.41300K_500_2500_2.10000V_0.00000T_Sep16-2014__16-49-14_001_091614.bin", "mod time(min)"=58229089.233333334, "file format"=enum."binary", "power(V)"=2.1, "Magn Field(T) "=0.0}, {"temperature"=163.066, "temperature str"="163.06600", "file path"=path "D:/Data/Ultrasound/LSCO/LSCO22__130814c/5_Cooling_2nd_try/September_2014/091614/163.06600K_500_2500_2.10000V_0.00000T_Sep16-2014__16-50-34_001_091614.bin", "last mod"=timestamp(3493745434 s since 1904-01-01), "file name str"="D:\\Data\\Ultrasound\\LSCO\\LSCO22__130814c\\5_Cooling_2nd_try\\September_2014\\091614\\163.06600K_500_2500_2.10000V_0.00000T_Sep16-2014__16-50-34_001_091614.bin", "mod time(min)"=58229090.56666667, "file format"=enum."binary", "power(V)"=2.1, "Magn Field(T) "=0.0}, {"temperature"=162.731, "temperature str"="162.73100", "file path"=path "D:/Data/Ultrasound/LSCO/LSCO22__130814c/5_Cooling_2nd_try/September_2014/091614/162.73100K_500_2500_2.10000V_0.00000T_Sep16-2014__16-51-53_001_091614.bin", "last mod"=timestamp(3493745513 s since 1904-01-01), "file name str"="D:\\Data\\Ultrasound\\LSCO\\LSCO22__130814c\\5_Cooling_2nd_try\\September_2014\\091614\\162.73100K_500_2500_2.10000V_0.00000T_Sep16-2014__16-51-53_001_091614.bin", "mod time(min)"=58229091.88333333, "file format"=enum."binary", "power(V)"=2.1, "Magn Field(T) "=0.0}, {"temperature"=162.385, "temperature str"="162.38500", "file path"=path "D:/Data/Ultrasound/LSCO/LSCO22__130814c/5_Cooling_2nd_try/September_2014/091614/162.38500K_500_2500_2.10000V_0.00000T_Sep16-2014__16-53-13_001_091614.bin", "last mod"=timestamp(3493745593 s since 1904-01-01), "file name str"="D:\\Data\\Ultrasound\\LSCO\\LSCO22__130814c\\5_Cooling_2nd_try\\September_2014\\091614\\162.38500K_500_2500_2.10000V_0.00000T_Sep16-2014__16-53-13_001_091614.bin", "mod time(min)"=58229093.21666667, "file format"=enum."binary", "power(V)"=2.1, "Magn Field(T) "=0.0}, {"temperature"=162.052, "temperature str"="162.05200", "file path"=path "D:/Data/Ultrasound/LSCO/LSCO22__130814c/5_Cooling_2nd_try/September_2014/091614/162.05200K_500_2500_2.10000V_0.00000T_Sep16-2014__16-54-32_001_091614.bin", "last mod"=timestamp(3493745672 s since 1904-01-01), "file name str"="D:\\Data\\Ultrasound\\LSCO\\LSCO22__130814c\\5_Cooling_2nd_try\\September_2014\\091614\\162.05200K_500_2500_2.10000V_0.00000T_Sep16-2014__16-54-32_001_091614.bin", "mod time(min)"=58229094.53333333, "file format"=enum."binary", "power(V)"=2.1, "Magn Field(T) "=0.0}, {"temperature"=161.701, "temperature str"="161.70100", "file path"=path "D:/Data/Ultrasound/LSCO/LSCO22__130814c/5_Cooling_2nd_try/September_2014/091614/161.70100K_500_2500_2.10000V_0.00000T_Sep16-2014__16-55-51_001_091614.bin", "last mod"=timestamp(3493745751 s since 1904-01-01), "file name str"="D:\\Data\\Ultrasound\\LSCO\\LSCO22__130814c\\5_Cooling_2nd_try\\September_2014\\091614\\161.70100K_500_2500_2.10000V_0.00000T_Sep16-2014__16-55-51_001_091614.bin", "mod time(min)"=58229095.85, "file format"=enum."binary", "power(V)"=2.1, "Magn Field(T) "=0.0}, {"temperature"=161.356, "temperature str"="161.35600", "file path"=path "D:/Data/Ultrasound/LSCO/LSCO22__130814c/5_Cooling_2nd_try/September_2014/091614/161.35600K_500_2500_2.10000V_0.00000T_Sep16-2014__16-57-11_001_091614.bin", "last mod"=timestamp(3493745831 s since 1904-01-01), "file name str"="D:\\Data\\Ultrasound\\LSCO\\LSCO22__130814c\\5_Cooling_2nd_try\\September_2014\\091614\\161.35600K_500_2500_2.10000V_0.00000T_Sep16-2014__16-57-11_001_091614.bin", "mod time(min)"=58229097.18333333, "file format"=enum."binary", "power(V)"=2.1, "Magn Field(T) "=0.0}, {"temperature"=161.021, "temperature str"="161.02100", "file path"=path "D:/Data/Ultrasound/LSCO/LSCO22__130814c/5_Cooling_2nd_try/September_2014/091614/161.02100K_500_2500_2.10000V_0.00000T_Sep16-2014__16-58-30_001_091614.bin", "last mod"=timestamp(3493745910 s since 1904-01-01), "file name str"="D:\\Data\\Ultrasound\\LSCO\\LSCO22__130814c\\5_Cooling_2nd_try\\September_2014\\091614\\161.02100K_500_2500_2.10000V_0.00000T_Sep16-2014__16-58-30_001_091614.bin", "mod time(min)"=58229098.5, "file format"=enum."binary", "power(V)"=2.1, "Magn Field(T) "=0.0}, {"temperature"=160.674, 
